vi "Send Data to Viewer Panel.vi"(9 "Message String":string, 10 "Topic Name":string, 11 "ViewerRef Array":T1[](array[typedef])) -> ()   [LabVIEW 2018]
uses:
  viewer/controls/viewewr_bus.ctl
  viewer/TopicViewer.lvlib
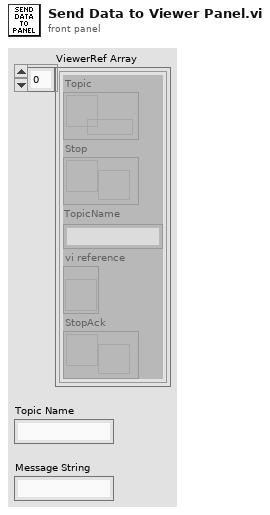
[diagram p1: front panel]
types:
  T1 = typedef "TopicViewer.lvlib/viewewr_bus.ctl" = cluster{"Topic":refnum<queue>, "Stop":refnum<notifier>, "TopicName":string, "vi reference":refnum<vi>, "StopAck":refnum<notifier>}
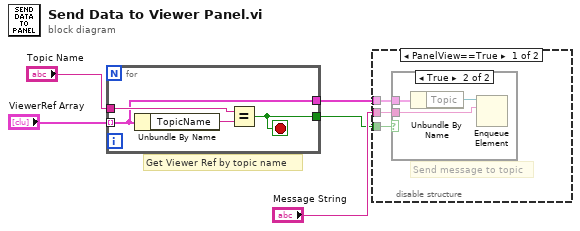
[diagram p0: block diagram]
diagram:
  # "Get Viewer Ref by topic name"
  n1 = for {
    tunnel: "ViewerRef Array" -> [w7] mode=indexing
    tunnel: "Topic Name" -> [w9]
    tunnel: [w7] -> w2
    tunnel: [w6] -> w3
    stop <- w6 stop-if-true
    n2 = Unbundle By Name(w7) -> ("TopicName"=w8:string)
    n3 = Equal?(x=w9, y=w8) -> (x = y?=w6:bool)
  }
  n4 = disable-structure shown="PanelView==True" {
    disable-tunnel: w2 -> [w12 _]
    disable-tunnel: w3 -> [w11 _]
    disable-tunnel: "Message String" -> [w10 _]
    frame condition #0 {
      # "Send message to topic"
      n5 = case shown="True" w11 {
        tunnel: w12 -> [_ w15]
        tunnel: w10 -> [_ w13]
        frame False {
        }
        frame True {
          n6 = Unbundle By Name(w15) -> ("Topic"=w14:refnum<queue>)
          n7 = Enqueue Element(queue=w14, element=w13) -> ()  [unwired: 2 in, 3 out]
        }
      }
    }
    frame condition #1 (active) {
    }
  }
